vi "ReadTangoTestShortAttributes.vi"() -> ()   [LabVIEW 2009]
uses:
  tango_lv8/tango_vi.llb/ReadShortScalarAttribute.vi
  tango_lv8/tango_vi.llb/ReadShortSpectrumAttribute.vi
  tango_lv8/tango_vi.llb/ReadShortImageAttribute.vi
panel:
  out "scalar attr. read (RO)":i16
  out "Read/s":dbl
  out "Read/s":dbl
  in  "?":bool=TRUE
  in  "?":bool=TRUE
  out "Read/s":dbl
  in  "?":bool=TRUE
  out "error stack":string[](array[string])
  out "error stack":string[](array[string])
  out "error stack":string[](array[string])
  out "scalar attr. value":i16(graph)
  out "scalar attr. write value":i16
  out "scalar attr. read value":i16
  out "?":bool
  in  "attr_name":string="short_scalar"
  out "?":bool
  in  "attr_name":string="short_spectrum_ro"
  out "?":bool
  out "image attr. value":i16[][](graph)
  out "spectrum attr. value":i16[](graph)
  in  "attr_name":string="short_image_ro"
  in  "dev_name":string="tango/tangotest/1"
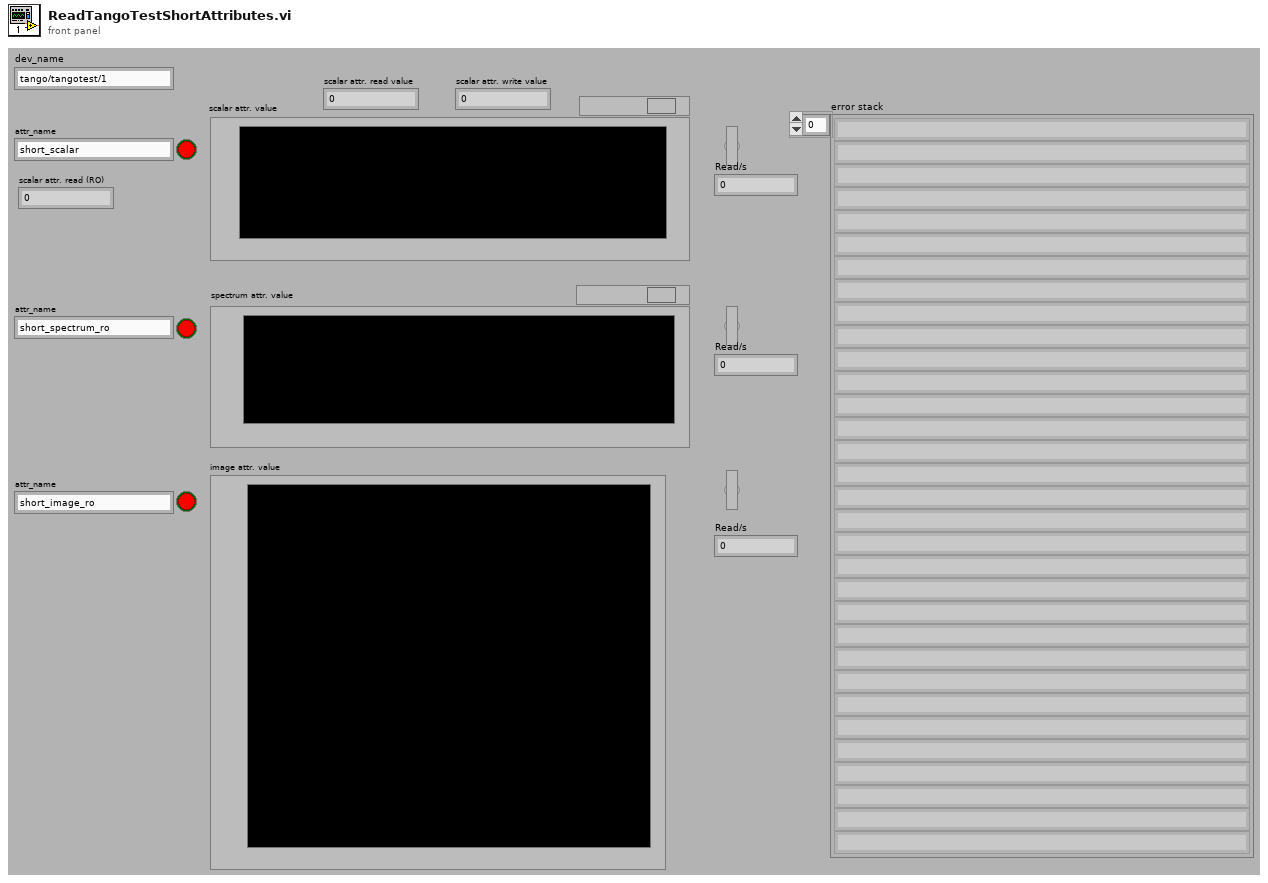
[diagram p1: front panel]
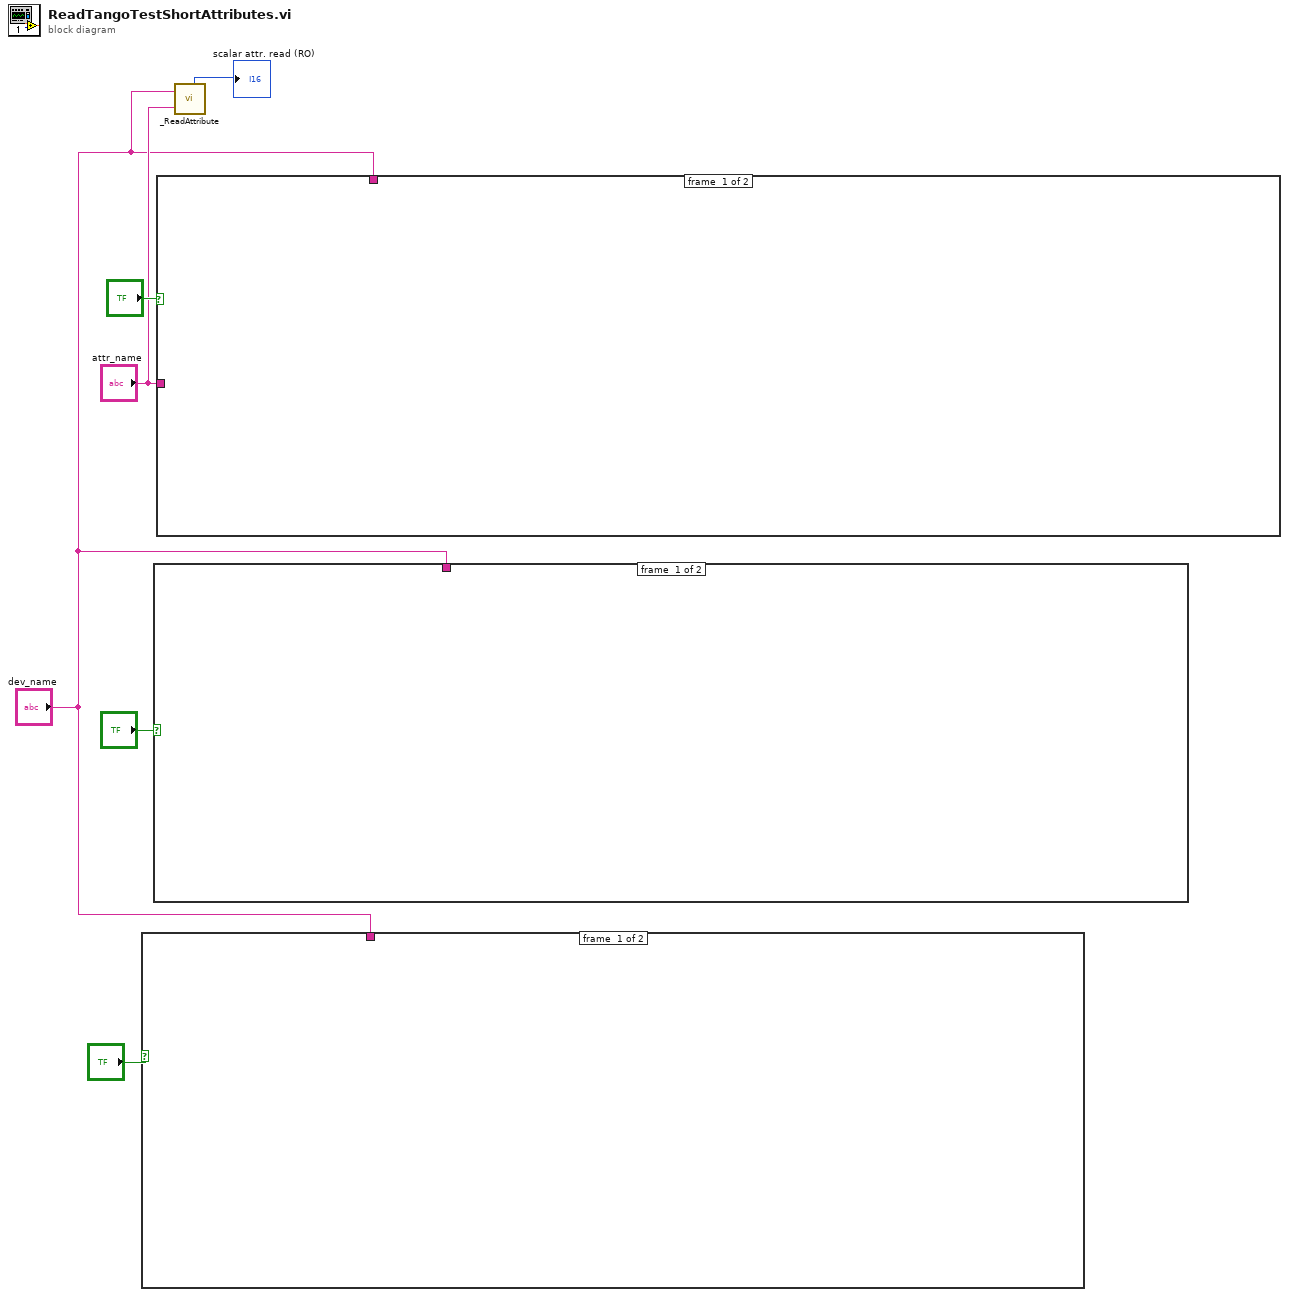
[diagram p0: block diagram]
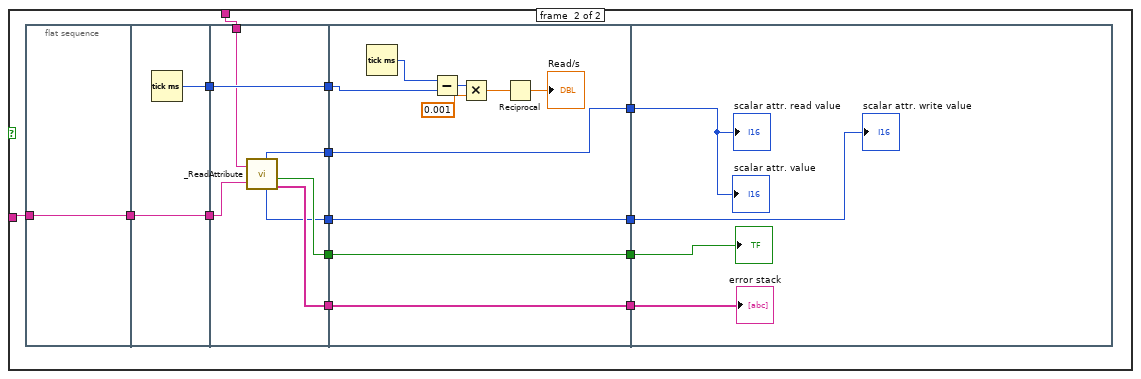
[diagram p2: hidden frame]
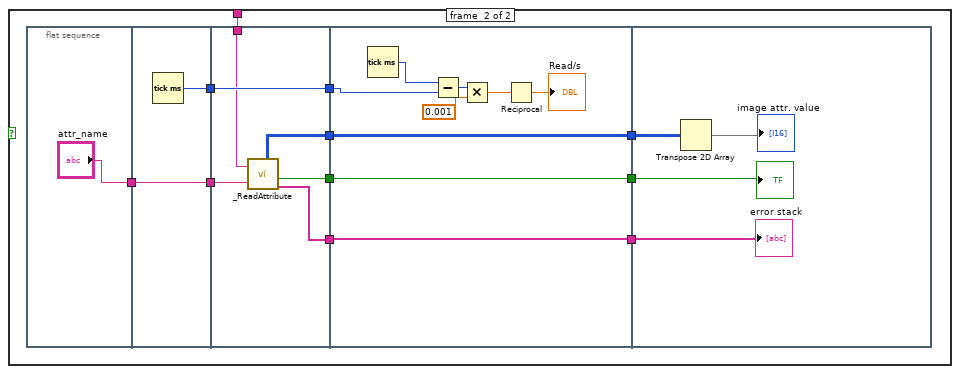
[diagram p3: hidden frame]
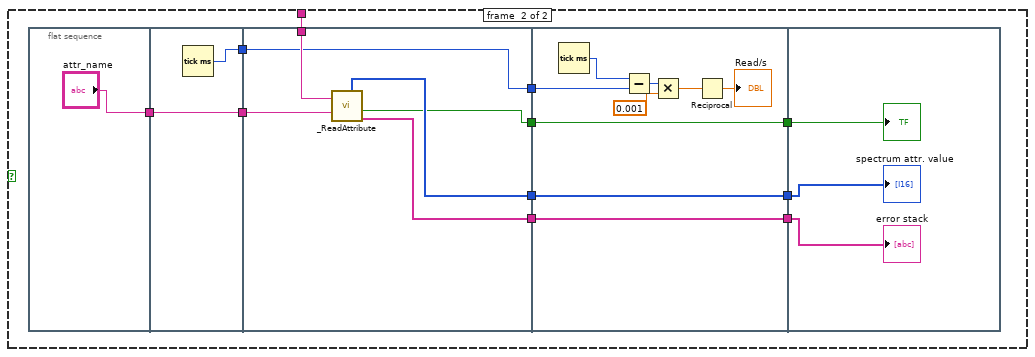
[diagram p4: hidden frame]
diagram:
  n1 = case shown="True" "?" {
    tunnel: "dev_name" -> [_ w11]
    frame #0 {
    }
    frame #1 {
      n2 = flat-sequence {
        tunnel: ["attr_name"] -> w16
        tunnel: [w20] -> w17
        tunnel: w16 -> [w20]
        tunnel: [w19] -> w15
        tunnel: w17 -> [w26]
        tunnel: w15 -> [w25]
        tunnel: [w25] -> w14
        tunnel: [w24] -> w12
        tunnel: w11 -> [w23]
        tunnel: [w22] -> w9
        tunnel: [w21] -> w7
        tunnel: w14 -> [w30]
        tunnel: [w29] -> w13
        tunnel: w12 -> [w29]
        tunnel: [w28] -> w10
        tunnel: w9 -> [w28]
        tunnel: [w27] -> w8
        tunnel: w7 -> [w27]
        tunnel: w13 -> [w36]
        tunnel: w10 -> [w38]
        tunnel: w8 -> [w37]
        frame #0 {
        }
        frame #1 {
          n3 = Tick Count (ms)() -> (millisecond timer value=w19:u32)
        }
        frame #2 {
          n4 = call-poly "_ReadAttribute.vi"("device name"=w23, "attribute name"=w26) -> ("value"=w22:i16[][], "success"=w21:bool, "error stack"=w24:string[])  [unwired: 3 out]
        }
        frame #3 {
          n5 = Tick Count (ms)() -> (millisecond timer value=w31:u32)
          n6 = Subtract(x=w31, y=w30) -> (x-y=w35:u32)
          n7 = Multiply(x=w35, y=0.001) -> (x*y=w32:dbl)
          n8 = Reciprocal(x=w32) -> (1/x=→"Read/s":dbl)
        }
        frame #4 {
          n9 = Transpose 2D Array(2D array=w38) -> (transposed array=→"image attr. value":i16[][])
          "?" <- w37
          "error stack" <- w36
        }
      }
    }
  }
  n10 = case shown="True" "?" {
    tunnel: "dev_name" -> [_ w42]
    frame #0 {
    }
    frame #1 {
      n11 = flat-sequence {
        tunnel: ["attr_name"] -> w50
        tunnel: [w53] -> w49
        tunnel: w50 -> [w53]
        tunnel: [w52] -> w48
        tunnel: w49 -> [w59]
        tunnel: w42 -> [w58]
        tunnel: w48 -> [w56]
        tunnel: [w55] -> w47
        tunnel: [w57] -> w46
        tunnel: [w56] -> w45
        tunnel: [w54] -> w40
        tunnel: [w66] -> w44
        tunnel: w47 -> [w66]
        tunnel: [w65] -> w43
        tunnel: w46 -> [w65]
        tunnel: w45 -> [w62]
        tunnel: [w60] -> w41
        tunnel: w40 -> [w60]
        tunnel: w44 -> [w70]
        tunnel: w43 -> [w71]
        tunnel: w41 -> [w69]
        frame #0 {
        }
        frame #1 {
          n12 = Tick Count (ms)() -> (millisecond timer value=w52:u32)
        }
        frame #2 {
          n13 = call-poly "_ReadAttribute.vi"("device name"=w58, "attribute name"=w59) -> ("value"=w55:i16[], "success"=w54:bool, "error stack"=w57:string[])  [unwired: 3 out]
        }
        frame #3 {
          n14 = Tick Count (ms)() -> (millisecond timer value=w63:u32)
          n15 = Subtract(x=w63, y=w62) -> (x-y=w68:u32)
          n16 = Multiply(x=w68, y=0.001) -> (x*y=w64:dbl)
          n17 = Reciprocal(x=w64) -> (1/x=→"Read/s":dbl)
        }
        frame #4 {
          "?" <- w69
          "spectrum attr. value" <- w70
          "error stack" <- w71
        }
      }
    }
  }
  n18 = case shown="True" "?" {
    tunnel: "dev_name" -> [_ w83]
    tunnel: "attr_name" -> [_ w74]
    frame #0 {
    }
    frame #1 {
      n19 = flat-sequence {
        tunnel: [w86] -> w75
        tunnel: w74 -> [w86]
        tunnel: [w88] -> w85
        tunnel: [w87] -> w76
        tunnel: w75 -> [w87]
        tunnel: w85 -> [w95]
        tunnel: [w95] -> w84
        tunnel: w83 -> [w91]
        tunnel: [w94] -> w81
        tunnel: [w93] -> w79
        tunnel: [w92] -> w77
        tunnel: w76 -> [w90]
        tunnel: [w89] -> w72
        tunnel: w84 -> [w100]
        tunnel: [w99] -> w82
        tunnel: w81 -> [w99]
        tunnel: [w98] -> w80
        tunnel: w79 -> [w98]
        tunnel: [w97] -> w78
        tunnel: w77 -> [w97]
        tunnel: [w96] -> w73
        tunnel: w72 -> [w96]
        tunnel: w82 -> [w106]
        tunnel: w80 -> [w109]
        tunnel: w78 -> [w108]
        tunnel: w73 -> [w107]
        frame #0 {
        }
        frame #1 {
          n20 = Tick Count (ms)() -> (millisecond timer value=w88:u32)
        }
        frame #2 {
          n21 = call-poly "_ReadAttribute.vi"("device name"=w91, "attribute name"=w90) -> ("value"=w94:i16, "setpoint"=w89:i16, "success"=w93:bool, "error stack"=w92:string[])  [unwired: 2 out]
        }
        frame #3 {
          n22 = Tick Count (ms)() -> (millisecond timer value=w101:u32)
          n23 = Subtract(x=w101, y=w100) -> (x-y=w105:u32)
          n24 = Multiply(x=w105, y=0.001) -> (x*y=w102:dbl)
          n25 = Reciprocal(x=w102) -> (1/x=→"Read/s":dbl)
        }
        frame #4 {
          "?" <- w109
          "scalar attr. read value" <- w106
          "scalar attr. value" <- w106
          "scalar attr. write value" <- w107
          "error stack" <- w108
        }
      }
    }
  }
  n26 = call-poly "_ReadAttribute.vi"("device name"="dev_name", "attribute name"="attr_name") -> ("value"=→"scalar attr. read (RO)":i16)  [unwired: 5 out]
